vi "Update Tuning from File.vi"(8 "error in (no error)":errorcluster, 11 "System Actor in":refnum<class "System Actor.lvclass">) -> (0 "error out":errorcluster, 1 "Tuning File":path, 2 "New Tuning File Created":bool, 3 "System Actor out":refnum<class "System Actor.lvclass">)   [LabVIEW 2014, in "Robot Actor Framework.lvlib" / "System Actor.lvlib" / "System Actor.lvclass"]
uses:
  System Actor.lvclass
  System Actor.lvclass/System Actor.ctl
  <vilib>/Utility/config.llb/NI_LVConfig.lvlib
  Utilities/Utilities.lvlib
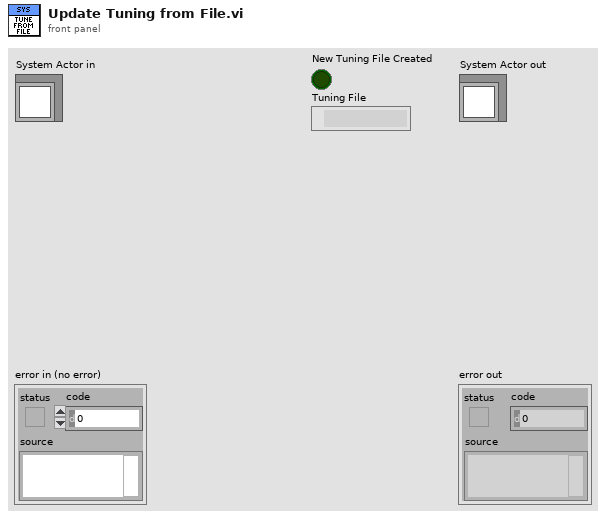
[diagram p1: front panel]
types:
  T1 = enum16{"Critical", "Error", "Warning", "Informational", "Debug"}
  T2 = typedef "Robot Actor Framework.lvlib/Trace.lvlib/Trace.lvclass/Trace Levels.ctl" = enum16{"Critical", "Error", "Warning", "Informational", "Debug"}
  T3 = typedef "NI_LVConfig.lvlib/Config Data RefNum.ctl" = refnum<k1>
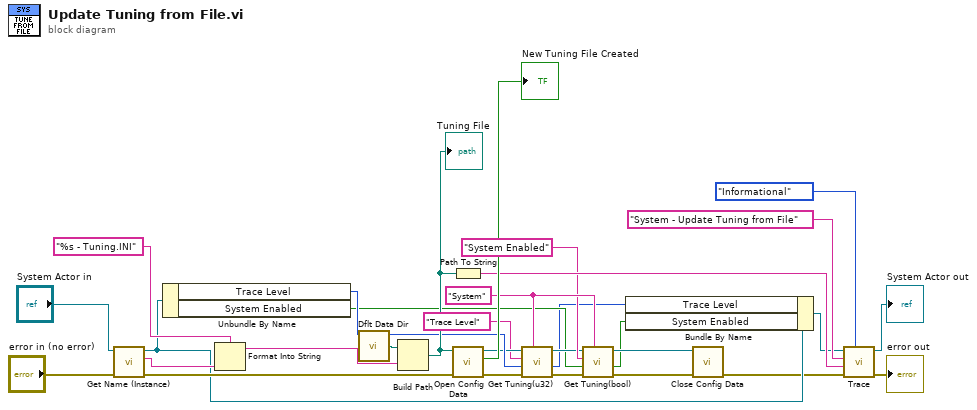
[diagram p0: block diagram]
diagram:
  w13 = "System" ("section")
  n1 = call-dynamic "Get Name (Instance).vi"("error in (no error)"="error in (no error)", "System Actor in"="System Actor in") -> ("error out"=w23:errorcluster, "System Name - Instance"=w27:string, "System Actor out"=w7:refnum<class "System Actor.lvclass">)  [unwired: 7 in]
  n2 = Unbundle By Name(w7) -> ("Trace Level"=w16:T2, "System Enabled"=w10:bool)
  n3 = Format Into String(format string="%s - Tuning.INI", w27) -> (resulting string=w26:string)  [unwired: 2 in, 1 out]
  n4 = call <vilib>:"Dflt Data Dir.vi"() -> ("App:Default Data Directory"=w30:path)
  n5 = Build Path(base path=w30, name or relative path=w26) -> (appended path=w19:path)
  "Tuning File" <- w19
  n6 = Path To String(path=w19) -> (string=w18:string)
  n7 = call <vilib>:"Open Config Data.vi"("error in (no error)"=w23, "configuration file path"=w19) -> ("error out"=w9:errorcluster, "file created?"=→"New Tuning File Created":bool, "refnum"=w15:T3)  [unwired: 7 in]
  n8 = call "Get Tuning(u32).vi"("section"=w13, "error in (no error)"=w9, "default value"=w16, "key"="Trace Level", "Config File refnum"=w15) -> ("error out"=w8:errorcluster, "value"=w2:u32, "Config File refnum out"=w11:T3)  [unwired: 4 in]
  n9 = call "Get Tuning(bool).vi"("section"=w13, "error in (no error)"=w8, "default value"=w10, "key"="System Enabled", "Config File refnum"=w11) -> ("error out"=w5:errorcluster, "value"=w1:bool, "Config File refnum out"=w6:T3)  [unwired: 4 in]
  n10 = Bundle By Name(cluster=w7, "Trace Level"=w2, "System Enabled"=w1) -> (w3:refnum<class "System Actor.lvclass">)
  n11 = call <vilib>:"Close Config Data.vi"("error in (no error)"=w5, "refnum"=w6) -> ("error out"=w4:errorcluster)  [unwired: 8 in, 1 out]
  n12 = call-dynamic "Trace.vi"("Trace Level"=T1."Informational", "error in (no error)"=w4, "System Message"=w18, "System Action"="System - Update Tuning from File", "System Actor in"=w3) -> ("error out"=→"error out":errorcluster, "System Actor out"=→"System Actor out":refnum<class "System Actor.lvclass">)  [unwired: 5 in]
